vi "Define Events.vi"(8 "error in (no error)":errorcluster, 11 "Example Controller in":refnum<class "Example Controller Actor.lvclass">) -> (0 "error out":errorcluster, 3 "Example Controller out":refnum<class "Example Controller Actor.lvclass">)   [LabVIEW 2023, in "Example Controller Actor.lvlib" / "Example Controller Actor.lvclass"]
doc: "This dynamic dispatch VI has to be overriden by the concrete Souce Actor subclasses in order to define the event served by the source"
uses:
  Example Controller Actor.lvclass
  Example Events/Double Array Event.lvclass
  Example Events/Timestamp Event.lvclass
  Example Events/Boolean Event.lvclass
  Example Controller Actor Messages/Update Boolean Event Msg/Update Boolean Event Msg.lvclass
  Event/Event.lvclass/Event.ctl
  Example Controller Actor.lvclass/Example Controller Actor.ctl
  Event/Event.lvclass
  Controller Actor/Controller Actor.lvclass
  C:/Projects/Shared Libraries/Event Actors/Examples/Timed Loop Controller/Timed Loop Controller/Timed Loop Controller.lvclass
  C:/Projects/Shared Libraries/Event Actors/Controller Actor/Controller Actor.lvclass
  C:/Program Files/National Instruments/LabVIEW 2023/vi.lib/ActorFramework/Actor/Actor.lvclass
  C:/Projects/Hardware Controller/Source/LSI Hardware Controller/View Interface/IView.lvclass
  C:/Projects/Shared Libraries/Event Actors/Examples/Example Controller Actor/Example Controller Actor/Example Controller Actor.lvclass
  C:/Projects/Shared Libraries/Event Actors/Event/Event.lvclass
  C:/Projects/Shared Libraries/Event Actors/Examples/Example Events/Double Array Event.lvclass
  C:/Projects/Shared Libraries/Event Actors/Examples/Example Events/Timestamp Event.lvclass
  C:/Projects/Shared Libraries/Event Actors/Event Data Types/Event Boolean/Event Boolean.lvclass
  C:/Projects/Shared Libraries/Event Actors/Examples/Example Events/Boolean Event.lvclass
  Example Events/Inited At Event.lvclass
  C:/Projects/Shared Libraries/Event Actors/Event Data Types/Event String/Event String.lvclass
  C:/Projects/Shared Libraries/Event Actors/Examples/Example Events/Inited At Event.lvclass
  C:/Projects/Shared Libraries/Event Actors/Event Handlers/Abstract Event Handler for Controller/Abstract Event Handler for Controller.lvclass
  C:/Projects/Shared Libraries/Event Actors/Examples/Example Controller Actor/Example Controller Actor Messages/Update Boolean Event Msg/Update Boolean Event Msg.lvclass
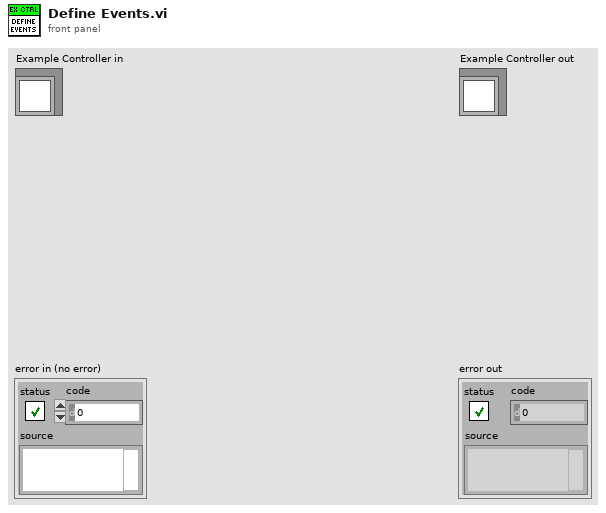
[diagram p1: front panel]
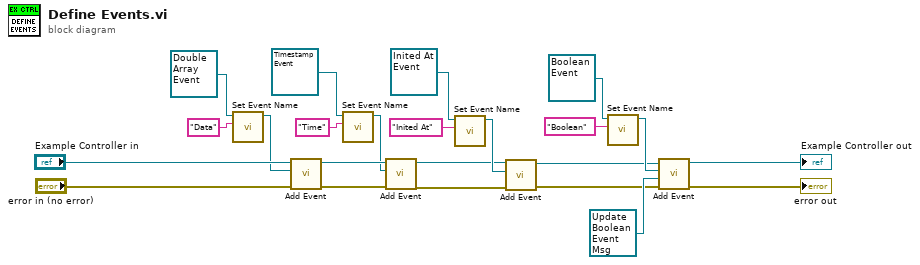
[diagram p0: block diagram]
diagram:
  n1 = call "Set Event Name.vi"("Name (Generic)"="Data", "Event In"=refnum<class "Double Array Event.lvclass"> refnum ("Double Array Event.lvclass")) -> ("Event Out"=w15:refnum<class "Double Array Event.lvclass">)  [unwired: 9 in]
  n2 = call "Add Event.vi"("error in (no error)"="error in (no error)", "Event"=w15, "Controller Actor in"="Example Controller in") -> ("error out"=w11:errorcluster, "Controller Actor out"=w16:refnum<class "Example Controller Actor.lvclass">)  [unwired: 7 in]
  n3 = call "Set Event Name.vi"("Name (Generic)"="Time", "Event In"=refnum<class "Timestamp Event.lvclass"> refnum ("Timestamp Event.lvclass")) -> ("Event Out"=w14:refnum<class "Timestamp Event.lvclass">)  [unwired: 9 in]
  n4 = call "Add Event.vi"("error in (no error)"=w11, "Event"=w14, "Controller Actor in"=w16) -> ("error out"=w4:errorcluster, "Controller Actor out"=w5:refnum<class "Example Controller Actor.lvclass">)  [unwired: 7 in]
  n5 = call "Set Event Name.vi"("Name (Generic)"="Inited At", "Event In"=refnum<class "Inited At Event.lvclass"> refnum ("Inited At Event.lvclass")) -> ("Event In"=w6:refnum<class "Inited At Event.lvclass">)  [unwired: 9 in]
  n6 = call "Add Event.vi"("error in (no error)"=w4, "Event"=w6, "Controller Actor in"=w5) -> ("error out"=w2:errorcluster, "Controller Actor in"=w3:refnum<class "Example Controller Actor.lvclass">)  [unwired: 7 in]
  n7 = call "Set Event Name.vi"("Name (Generic)"="Boolean", "Event In"=refnum<class "Boolean Event.lvclass"> refnum ("Example Source.lvlib:Boolean Event.lvclass")) -> ("Event Out"=w13:refnum<class "Boolean Event.lvclass">)  [unwired: 9 in]
  n8 = call "Add Event.vi"("error in (no error)"=w2, "Controller Event Fire Handler"=refnum<class "Update Boolean Event Msg.lvclass"> refnum ("Example Source.lvlib:Update Boolean Msg.lvclass"), "Event"=w13, "Controller Actor in"=w3) -> ("error out"=→"error out":errorcluster, "Controller Actor out"=→"Example Controller out":refnum<class "Example Controller Actor.lvclass">)  [unwired: 6 in]
